vi "copy excel template.vi"(8 "error in (no error)":errorcluster, 10 "report file path in":path, 11 "template file path in":path) -> (0 "error out":errorcluster, 2 "report file path out":path)   [LabVIEW 2016]
uses:
  <vilib>/Utility/NIReport.llb/NI_report.lvclass
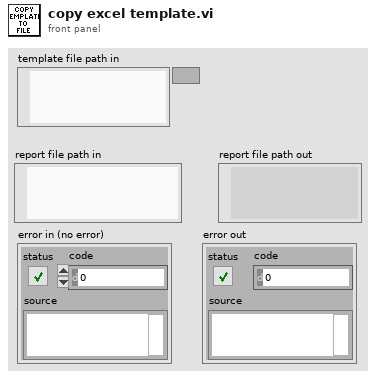
[diagram p1: front panel]
types:
  T1 = enum16{"maximized", "minimized", "normal", "no change"}
  T2 = enum16{"Standard Report", "HTML", "Word", "Excel"}
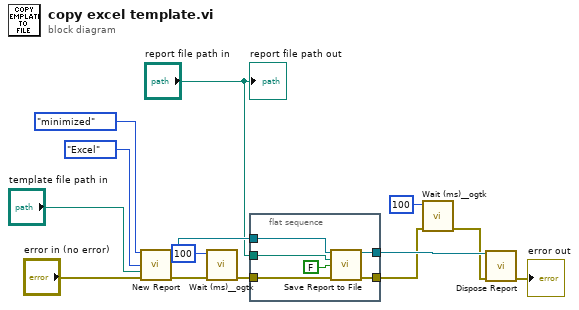
[diagram p0: block diagram]
diagram:
  n1 = call <vilib>:"New Report.vi"("window state (normal)"=T1."minimized", "report type"=T2."Excel", "template (empty)"="template file path in", "error in (no error)"="error in (no error)") -> ("report out"=w7:refnum<class "NI_report.lvclass">, "error out"=w9:errorcluster)  [unwired: 10 in]
  n2 = call <userlib>:"Wait (ms)__ogtk.vi"("error in (no error)"=w9, "milliseconds to wait"=u32 100) -> ("error out"=w6:errorcluster)  [unwired: 8 in, 1 out]
  n3 = flat-sequence {
    tunnel: [w20] -> w5
    tunnel: [w19] -> w3
    tunnel: w6 -> [w17]
    tunnel: w7 -> [w16]
    tunnel: "report file path in" -> [w15]
    frame #0 {
      n4 = call-dynamic "Save Report to File.vi"("report in"=w16, "report file path"=w15, "prompt to replace? (F)"=FALSE, "error in (no error)"=w17) -> ("report out"=w20:refnum<class "NI_report.lvclass">, "error out"=w19:errorcluster)  [unwired: 10 in]
    }
  }
  n5 = call <userlib>:"Wait (ms)__ogtk.vi"("error in (no error)"=w3, "milliseconds to wait"=u32 100) -> ("error out"=w2:errorcluster)  [unwired: 8 in, 1 out]
  n6 = call-dynamic "Dispose Report.vi"("report in"=w5, "error in (no error)"=w2) -> ("error out"=→"error out":errorcluster)  [unwired: 13 in]
  "report file path out" <- "report file path in"
